vi "PS Read.vi"(8 "error in (no error)":errorcluster, 9 "Message Data":variant, 10 "XYZ notifier":refnum<notifier>, 11 "Hardware Resources in":T1={"Tango HW"={"VISA resource"="", "Baud Rate (115200)"=2, "lAnInterfaceType"=0, "bAShowProt"=15}, "Writer Queue"=refnum, "Status"=FALSE, "Abs Position"=[], "Axis Velocity"={"dX"=0.0, "dY"=0.0, "dZ"=0.0, "dA"=0.0}, "acceleration "=0.0, "Z direction"=enum."Up", "Position Mode"="", "plLSID"=0}) -> (0 "error out":errorcluster, 1 "Message Data Out":variant, 3 "Hardware Resources out":T1={"Tango HW"={"VISA resource"="", "Baud Rate (115200)"=2, "lAnInterfaceType"=0, "bAShowProt"=15}, "Writer Queue"=refnum, "Status"=FALSE, "Abs Position"=[], "Axis Velocity"={"dX"=0.0, "dY"=0.0, "dZ"=0.0, "dA"=0.0}, "acceleration "=0.0, "Z direction"=enum."Up", "Position Mode"="", "plLSID"=0})   [LabVIEW 2020, in "MOTOR.lvlib"]
doc: "Perform the acquisition. Replace the contents of this diagram with calls to acquisition hardware."
uses:
  MOTOR.lvlib
  PS Hardware Configuration.ctl
  support/Message Queue/Message Cluster.ctl
  support/Message Queue/Message Queue.lvlib
  <instrlib>/Tango_DLL/Tango_DLL.lvlib
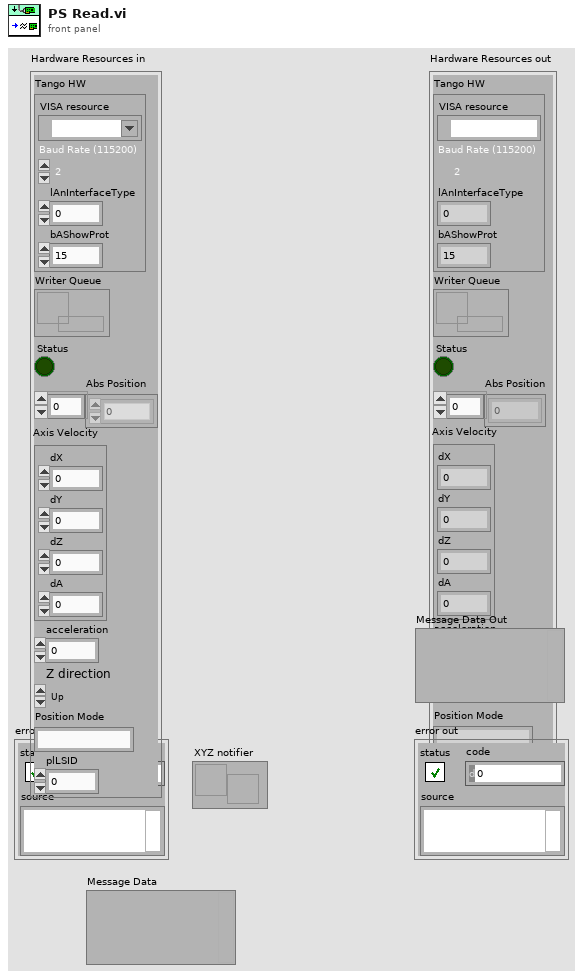
[diagram p1: front panel]
types:
  T1 = typedef "MOTOR.lvlib/PS Hardware Configuration.ctl" = cluster{"Tango HW":cluster{"VISA resource":refnum<visa-resource-name>, "Baud Rate (115200)":i32, "lAnInterfaceType":i32, "bAShowProt":i32}, "Writer Queue":refnum<queue>, "Status":bool, "Abs Position":i32[], "Axis Velocity":cluster{"dX":dbl, "dY":dbl, "dZ":dbl, "dA":dbl}, "acceleration ":dbl, "Z direction":enum16{"Up", "Down"}, "Position Mode":string, "plLSID":i32}
  T2 = typedef "Message Queue.lvlib/Message Cluster.ctl" = cluster{"Message":string, "Message Data":variant}
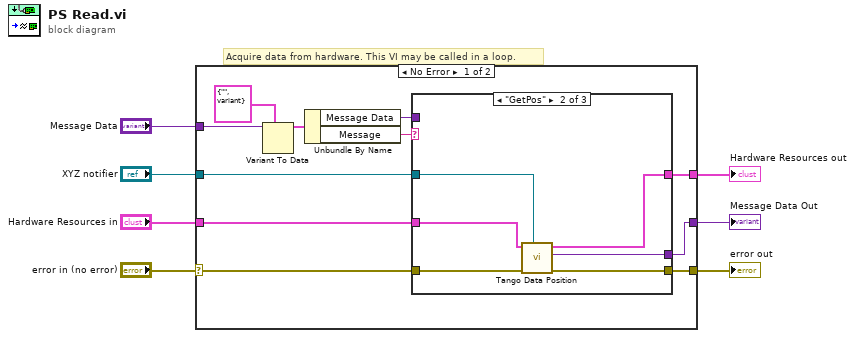
[diagram p0: block diagram]
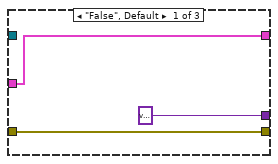
[diagram p2: hidden frame]
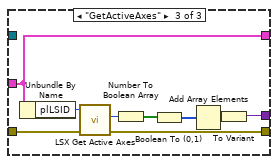
[diagram p3: hidden frame]
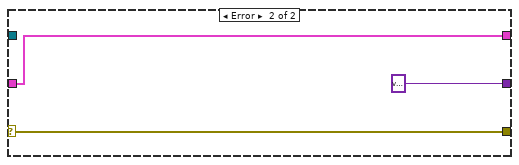
[diagram p4: hidden frame]
diagram:
  # "Acquire data from hardware. This VI may be called in a loop."
  n1 = case shown="No Error" "error in (no error)" {
    selector: "error in (no error)" -> [w18 w37]
    tunnel: [w15 w37] -> w6
    tunnel: "Hardware Resources in" -> [w17 w38]
    tunnel: [w16 w38] -> w4
    tunnel: [w14 variant ("Message Data Out")] -> w3
    tunnel: "XYZ notifier" -> [w11 _]
    tunnel: "Message Data" -> [w10 _]
    frame No Error {
      n2 = Variant To Data(type=T2 {"Message"="", "Message Data"=variant} ("element"), Variant=w10) -> (data=w12:T2)  [unwired: 1 in, 1 out]
      n3 = Unbundle By Name(w12) -> ("Message Data"=w8:variant, "Message"=w9:string)
      n4 = case shown="\"GetPos\"" w9 {
        tunnel: w18 -> [w20 w27 w35]
        tunnel: w17 -> [w21 w26 w34]
        tunnel: [w21 w25 w34] -> w16
        tunnel: [w20 w24 w35] -> w15
        tunnel: [variant ("Message Data Out") w23 w28] -> w14
        tunnel: w11 -> [_ w22 _]
        tunnel: w8 -> [_ _ _]
        frame "False", Default {
        }
        frame "GetPos" {
          n5 = call "Tango Data Position.vi"("XYZ notifier"=w22, "error in (no error)"=w27, "Hardware Resources in"=w26) -> ("error out"=w24:errorcluster, "Message Data Out"=w23:variant, "Hardware Resources out"=w25:T1)  [unwired: 6 in]
        }
        frame "GetActiveAxes" {
          n6 = Unbundle By Name(w34) -> ("plLSID"=w33:i32)
          n7 = call <instrlib>:"LSX Get Active Axes.vi"("lLSID"=w33) -> ("plFlags out"=w32:i32)  [unwired: 8 in, 2 out]
          n8 = Number To Boolean Array(number=w32) -> (Boolean array=w31:bool[])
          n9 = Boolean To (0,1)(Boolean=w31) -> (0, 1=w30:i16[])
          n10 = Add Array Elements(numeric array=w30) -> (sum=w29:i16)
          n11 = To Variant(anything=w29) -> (Variant=w28:variant)
        }
      }
    }
    frame Error {
    }
  }
  "Hardware Resources out" <- w4
  "error out" <- w6
  "Message Data Out" <- w3
